vi "ziModClear.vi"(7 "Error In":errorcluster, 10 "ziModHandle In":T1 {"ModHandle" format="0x%08x"; "Conn" format="0x%08x"}) -> (0 "Error Out":errorcluster, 3 "ModHandle Out":T1 {"ModHandle" format="0x%08x"; "Conn" format="0x%08x"})   [LabVIEW 2015, in "Zurich Instruments LabOne.lvlib"]
doc: "Destroys a module."
uses:
  Zurich Instruments LabOne.lvlib
  Zurich Instruments/LabOne/API/LabVIEW/Zurich Instruments LabOne/Private/ziLV64.framework
  ziTypeModHandle.ctl
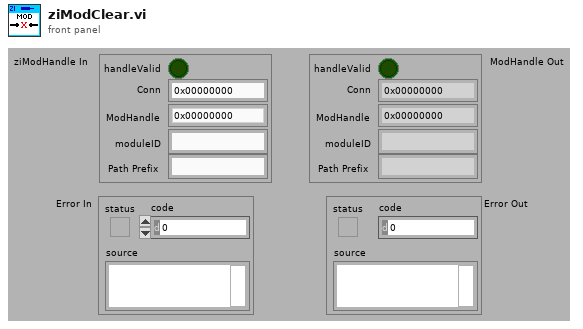
[diagram p1: front panel]
types:
  T1 = typedef "Zurich Instruments LabOne.lvlib/ziTypeModHandle.ctl" = cluster{"handleValid":bool, "Conn":u64, "ModHandle":u64, "moduleID":string, "Path Prefix":string}
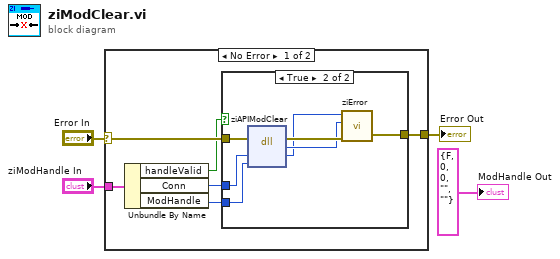
[diagram p0: block diagram]
diagram:
  n1 = case shown="No Error" "Error In" {
    selector: "Error In" -> [w9 w19]
    tunnel: "ziModHandle In" -> [w8 _]
    tunnel: [w10 w19] -> w4
    frame No Error {
      n2 = Unbundle By Name(w8) -> ("handleValid"=w7:bool, "Conn"=w6:u64, "ModHandle"=w5:u64)
      n3 = case shown="True" w7 {
        tunnel: w9 -> [w11 w18]
        tunnel: [w11 w15] -> w10
        tunnel: w6 -> [_ w14]
        tunnel: w5 -> [_ w13]
        frame False {
        }
        frame True {
          n4 = dll-call lib="Users/arkady/Desktop/ado/github/resonant_ultrasound_arxiv/maglab ultrasound -- arkady --arxiv/Zurich Instruments/LabOne/API/LabVIEW/Zurich Instruments LabOne/Private/ziLV*.*" fn="ziAPIModClear"(error in=w18, "conn"=w14, "ModHandle"=w13) -> (error out=w17:errorcluster, "return type"=w16:u32, "conn"=w12:u64)  [unwired: 3 in, 1 out]
          n5 = call "ziError.vi"("Conn"=w12, "ziErrorCode"=w16, "Error In"=w17) -> ("Error Out"=w15:errorcluster)  [unwired: 2 in, 1 out]
        }
      }
    }
    frame Error {
    }
  }
  "Error Out" <- w4
  "ModHandle Out" <- T1 {"handleValid"=FALSE, "Conn"=0, "ModHandle"=0, "moduleID"="", "Path Prefix"=""} ("ModHandle Out")
